vi "Get Error (Logic).vi"(8 "error in (no error)":errorcluster, 11 "Error (Logic)Ref":refnum<vi>) -> (0 "error out":errorcluster)   [LabVIEW 2025, in "I2C Bus Monitor UI.lvlib"]
uses:
  I2C Bus Monitor UI.lvlib
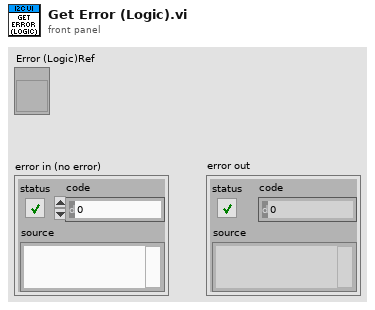
[diagram p1: front panel]
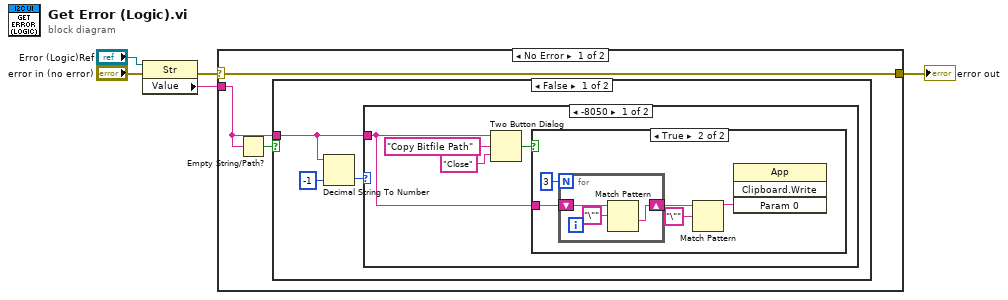
[diagram p0: block diagram]
diagram:
  n1 = property class="Str"(reference="Error (Logic)Ref", error in="error in (no error)") -> (error out=w3:errorcluster, "Value"=w2:string)  [unwired: 1 out]
  n2 = case shown="No Error" w3 {
    selector: w3 -> [w8 w24]
    tunnel: w2 -> [w6 _]
    tunnel: [w8 w24] -> w1
    frame No Error {
      n3 = Empty String/Path?(string/path=w6) -> (empty?=w7:bool)
      n4 = case shown="False" w7 {
        tunnel: w6 -> [w11 _]
        frame False {
          n5 = Decimal String To Number(string=w11, default (0L)=-1 ("default (0 I32)")) -> (number=w9:i32)  [unwired: 1 in, 1 out]
          n6 = case shown="-8050" w9 {
            tunnel: w11 -> [w13 _]
            frame -8050 {
              n7 = Two Button Dialog(message=w13, 1:"Close" ("F button name (\"Cancel\")"), 2:"Copy Bitfile Path" ("T button name (\"OK\")")) -> (T button?=w14:bool)
              n8 = case shown="True" w14 {
                tunnel: w13 -> [_ w20]
                frame False {
                }
                frame True {
                  n9 = for {
                    N: 3 -> [_]
                    shift-right: [w21] -> w18
                    shift-left: w20 -> [w23]
                    n10 = Match Pattern(string=w23, regular expression="\"") -> (after substring=w21:string)  [unwired: 1 in, 3 out]
                  }
                  n11 = Match Pattern(string=w18, regular expression="\"") -> (before substring=w16:string)  [unwired: 1 in, 3 out]
                  n12 = invoke class="App" method="Clipboard.Write"("Param 0"=w16) -> ()  [unwired: 3 in, 4 out]
                }
              }
            }
            frame -1, Default {
            }
          }
        }
        frame True {
        }
      }
    }
    frame Error {
    }
  }
  "error out" <- w1
